vi "End.vi"(8 "error in (no error)":errorcluster, 11 "SPARC4_GUI in":refnum<class "SPARC4_GUI.lvclass">) -> (0 "error out":errorcluster, 3 "SPARC4_GUI out":refnum<class "SPARC4_GUI.lvclass">)   [LabVIEW 2018, in "SPARC4_GUI.lvclass"]
uses:
  SPARC4_GUI.lvclass
  SPARC4_GUI.lvclass/SPARC4_GUI.ctl
  Channel GUI/Channel GUI.lvclass
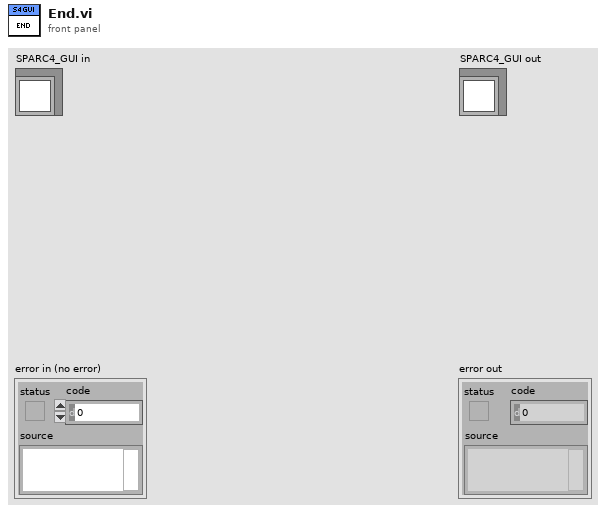
[diagram p1: front panel]
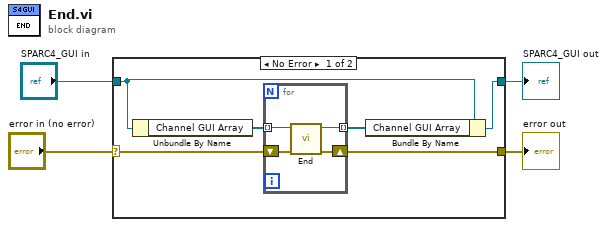
[diagram p0: block diagram]
diagram:
  n1 = case shown="No Error" "error in (no error)" {
    selector: "error in (no error)" -> [w8 w16]
    tunnel: [w7 w16] -> w3
    tunnel: [w9 w15] -> w1
    tunnel: "SPARC4_GUI in" -> [w10 w15]
    frame No Error {
      n2 = Unbundle By Name(w10) -> ("Channel GUI Array"=w5:refnum<class "Channel GUI.lvclass">[])
      n3 = for {
        tunnel: [w12] -> w6 mode=indexing
        tunnel: w5 -> [w11] mode=indexing
        shift-right: [w13] -> w7
        shift-left: w8 -> [w14]
        n4 = call "End.vi"("error in (no error)"=w14, "Channel GUI in"=w11) -> ("error out"=w13:errorcluster, "Channel GUI out"=w12:refnum<class "Channel GUI.lvclass">)  [unwired: 8 in]
      }
      n5 = Bundle By Name(cluster=w10, "Channel GUI Array"=w6) -> (w9:refnum<class "SPARC4_GUI.lvclass">)
    }
    frame Error {
    }
  }
  "error out" <- w3
  "SPARC4_GUI out" <- w1
